vi "Read Long Parameter.vi"(7 "process number":u8, 8 "error in (no error)":errorcluster, 9 "parameter number":u8, 10 "node address (same)":u8, 11 "ProPar in":refnum<class "PL Bronkhorst ProPar.lvclass">) -> (0 "error out":errorcluster, 2 "value":u32, 3 "ProPar out":refnum<class "PL Bronkhorst ProPar.lvclass">)   [LabVIEW 2015, in "PL Bronkhorst ProPar.lvclass"]
doc: "Reads specified long <b>parameter</b> of the specified <b>node</b>."
uses:
  PL Bronkhorst ProPar.lvclass
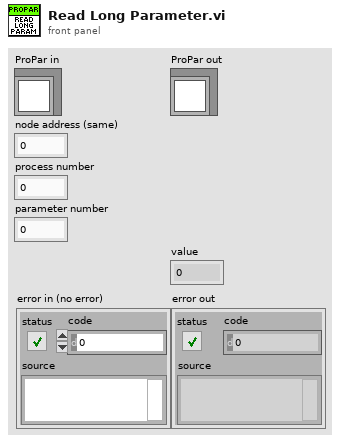
[diagram p1: front panel]
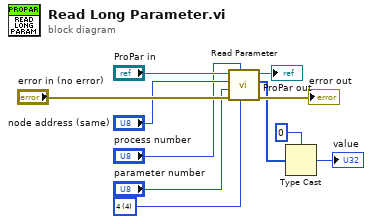
[diagram p0: block diagram]
diagram:
  w1 = u8 4 items=["variable"=0, "1"=1, "2"=2, "4"=4] ("value byte count (variable)")
  n1 = call "Read Parameter.vi"("value byte count"=w1, "process number"="process number", "error in (no error)"="error in (no error)", "parameter number"="parameter number", "node address (same)"="node address (same)", "ProPar in"="ProPar in") -> ("error out"=→"error out":errorcluster, "value"=w4:u8[], "ProPar out"=→"ProPar out":refnum<class "PL Bronkhorst ProPar.lvclass">)  [unwired: 3 in]
  n2 = Type Cast(type=u32 0 ("value"), x=w4) -> (*(type *) &x=→"value":u32)
